vi "add many tags.vi"(10 "tags":T1[](array[typedef]), 11 "EIP Tags Configuration in":refnum<class "EIP Tags Configuration.lvclass">) -> (0 "error out":errorcluster, 2 "Array":T1[](array[typedef]), 3 "EIP Tags Configuration out":refnum<class "EIP Tags Configuration.lvclass">)   [LabVIEW 2013, in "EIP Tags editor node.lvclass"]
uses:
  EIP Tags editor node.lvclass
  <vilib>/NI/TBM Modules/EIP Tags/configuration/eip tag definition.ctl
  <vilib>/NI/TBM Modules/EIP Tags/configuration/eip tag types.ctl
  <vilib>/NI/TBM Modules/EIP Tags/configuration/EIP Tags Configuration.lvclass
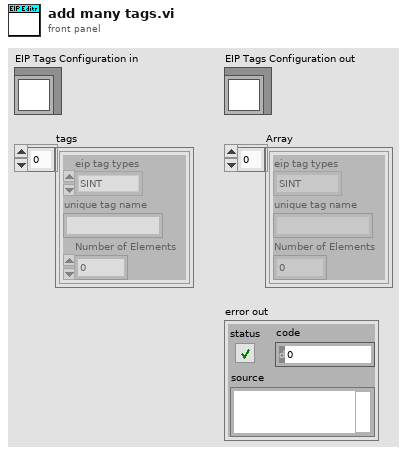
[diagram p1: front panel]
types:
  T1 = typedef "EIP Tags Configuration.lvclass/eip tag definition.ctl" = cluster{"eip tag types":T2, "unique tag name":string, "Number of Elements":u32}
  T2 = typedef "EIP Tags Configuration.lvclass/eip tag types.ctl" = enum16{"SINT", "INT", "DINT", "REAL", "BOOL", "STRING"}
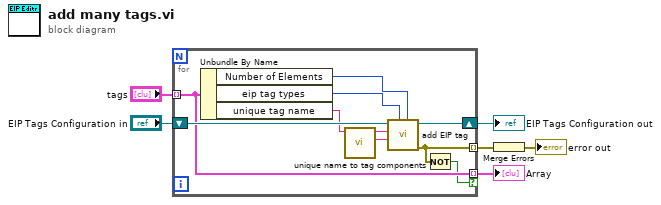
[diagram p0: block diagram]
diagram:
  n1 = for {
    tunnel: [w7] -> w1 mode=indexing
    tunnel: "tags" -> [w9] mode=indexing
    shift-right: [w16] -> w2
    shift-left: "EIP Tags Configuration in" -> [w15]
    tunnel: [w9] -> w6 mode=indexing if=w8
    n2 = Unbundle By Name(w9) -> ("Number of Elements"=w13:u32, "eip tag types"=w14:T2, "unique tag name"=w12:string)
    n3 = call <vilib>:"unique name to tag components.vi"("unique name"=w12) -> ("Tag Name"=w10:string, "Network Path"=w11:string)  [unwired: 9 in]
    n4 = call <vilib>:"add EIP tag.vi"("Number of Elements"=w13, "eip tag types"=w14, "Tag Name"=w10, "Network Path"=w11, "EIP Tags configuration in"=w15) -> ("error out"=w7:errorcluster, "EIP Tags configuration out"=w16:refnum<class "EIP Tags Configuration.lvclass">)  [unwired: 5 in]
    n5 = Not(x=w7) -> (.not. x?=w8:bool)
  }
  "Array" <- w6
  "EIP Tags Configuration out" <- w2
  n6 = Merge Errors(w1) -> (→"error out":errorcluster)
